vi "optimization2_secondround.vi"() -> ()   [LabVIEW 2020]
uses:
  <vilib>/gmath/GlobalOptimization.llb/DE_Stopping Criteria.ctl
  <vilib>/gmath/GlobalOptimization.llb/DE_Settings.ctl
  <vilib>/gmath/GlobalOptimization.llb/DE_Bound Mapping Method.ctl
  <vilib>/gmath/GlobalOptimization.llb/DE_Mutation Method.ctl
  <vilib>/gmath/GlobalOptimization.llb/DE_Crossover Method.ctl
  <vilib>/gmath/NI_AAL_GlobalOptimization.lvlib
panel:
  in  "Image acquisition time (ms)":dbl=976.0
  in  "Flyback time (ms)":dbl=24.0
  out "Minimum":dbl[](array[numeric])=[0.4292106274702698, 0.5476138169757999, -0.05543112551298741, -0.011925036985674273]
  out "F(Minimum)":dbl[](array[numeric])=[4.960999229893729]
  in  "DE settings":T1={"population size"=10, "scale factor"=0.9, "crossover probability"=0.95, "bound mapping method"=1, "mutation method"=0, "crossover method"=0} {"crossover method" items=["Uniform", "Exponential"]; "mutation method" items=["Random", "Either Or", "Best", "Target to Best"]; "bound mapping method" items=["None", "Random between Bounds and Values", "Re-Initialize"]}
  in  "stopping criteria":T5={"max iterations"=10, "max function calls"=-1, "max time (sec)"=-1.0}
  out "number of function calls":i32=110
  in  "Bounds":cluster{"Min":dbl[], "Max":dbl[]}={"Min"=[-2.761, 0.192, 3.211, -0.299, 115.9, -108.5, 0.642], "Max"=[-2.751, 0.194, 3.231, -0.291, 117.0, -107.9, 0.645]}
  out "VI Type":T6(ring)=enum."Standard VI"
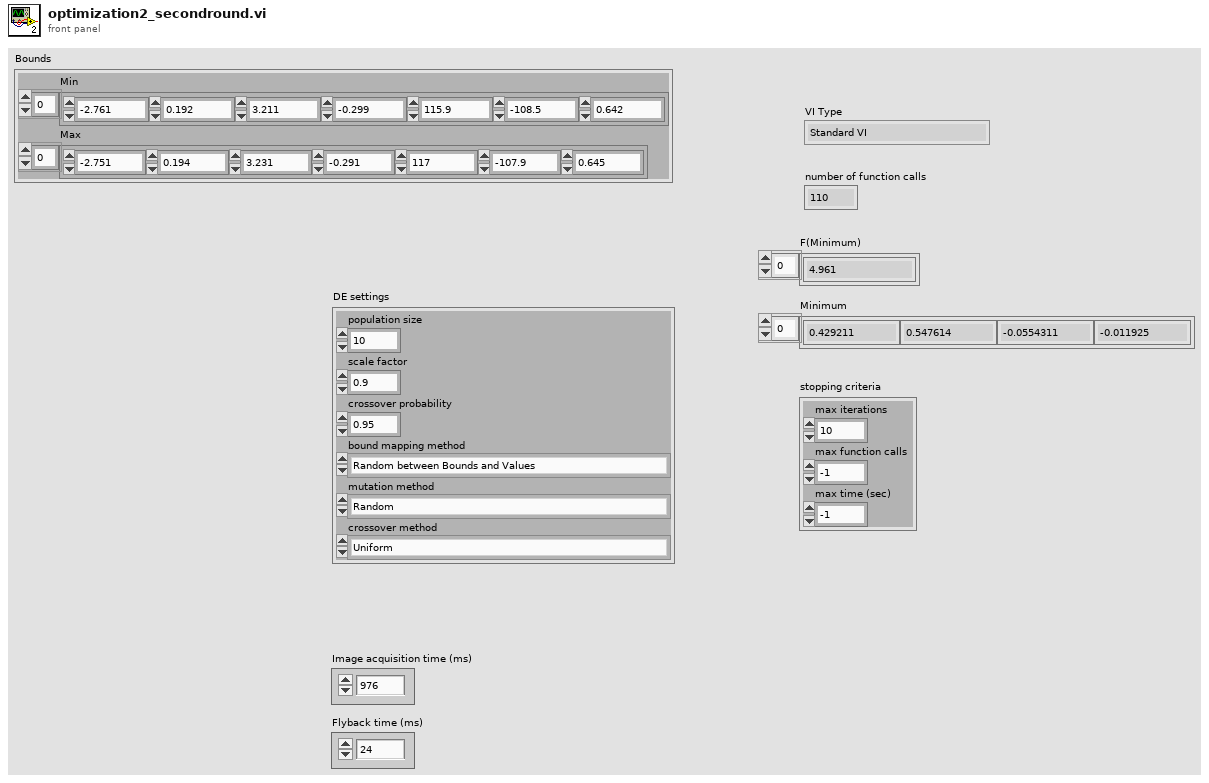
[diagram p1: front panel]
types:
  T1 = typedef "NI_AAL_GlobalOptimization.lvlib/DE_Settings.ctl" = cluster{"population size":i32, "scale factor":dbl, "crossover probability":dbl, "bound mapping method":T2, "mutation method":T3, "crossover method":T4}
  T2 = typedef "NI_AAL_GlobalOptimization.lvlib/DE_Bound Mapping Method.ctl" = u16
  T3 = typedef "NI_AAL_GlobalOptimization.lvlib/DE_Mutation Method.ctl" = u16
  T4 = typedef "NI_AAL_GlobalOptimization.lvlib/DE_Crossover Method.ctl" = u16
  T5 = typedef "NI_AAL_GlobalOptimization.lvlib/DE_Stopping Criteria.ctl" = cluster{"max iterations":i32, "max function calls":i32, "max time (sec)":dbl}
  T6 = enum32{"invalid VI type", "Standard VI", "Control VI", "Global VI", "Polymorphic VI", "Configuration VI", "SubSystem", "Facade VI", "Method VI", "Statechart Diagram VI"}
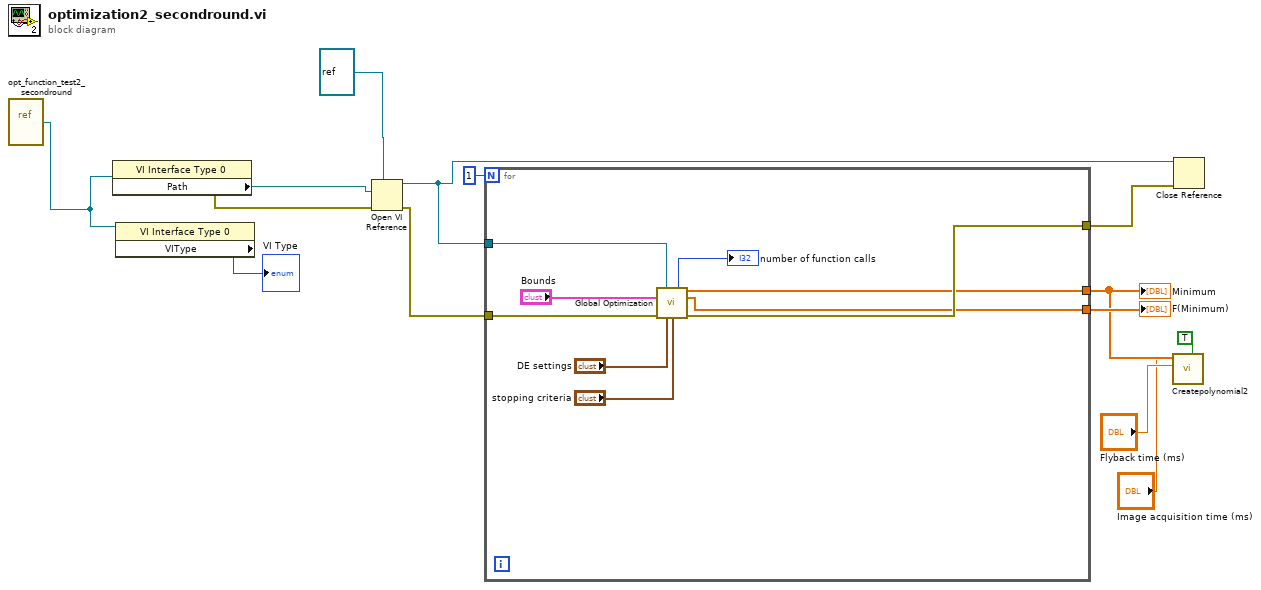
[diagram p0: block diagram]
diagram:
  n1 = vi-ref "opt_function_test2_secondround.vi"() -> (w2:refnum<vi>)
  n2 = property class="VI Interface Type 0"(reference=w2) -> (error out=w4:errorcluster, "Path"=w5:path)  [unwired: 1 in, 1 out]
  n3 = property class="VI Interface Type 0"(reference=w2) -> ("VIType"=→"VI Type":T6)  [unwired: 1 in, 2 out]
  n4 = Open VI Reference(type specifier VI Refnum (for type only)=refnum<vi> refnum, vi path=w5, error in (no error)=w4) -> (vi reference=w3:refnum<vi>, error out=w11:errorcluster)  [unwired: 3 in]
  n5 = for {
    N: 1 -> [_]
    tunnel: [w19] -> w12
    tunnel: w11 -> [w18]
    tunnel: [w17] -> w9
    tunnel: [w16] -> w10
    tunnel: w3 -> [w15]
    n6 = call <vilib>:"Global Optimization.vi"("objective and constraint function"=w15, "Bounds"="Bounds", "error in (no error)"=w18, "DE settings"="DE settings", "stopping criteria"="stopping criteria") -> ("number of function calls"=→"number of function calls":i32, "Minimum"=w17:dbl[], "F(Minimum)"=w16:dbl[], "error out"=w19:errorcluster)  [unwired: 6 in, 1 out]
  }
  "F(Minimum)" <- w10
  "Minimum" <- w9
  n7 = call "Createpolynomial2.vi"("Flyback (ms)"="Flyback time (ms)", "Acquisition time (ms)"="Image acquisition time (ms)", "Save calibration"=TRUE, "P(x)"=w9) -> ()  [unwired: 7 in, 1 out]
  n8 = Close Reference(reference=w3, error in (no error)=w12) -> ()  [unwired: 1 out]
